vi "emi_Error Filter Single.vi"(1 "Action(No Error)":T2, 5 "Error Code":i32, 9 "error in (no error)":errorcluster, 12 "Filter(Error&Warning)":T1) -> (8 "Filter Triggered":bool, 10 "error out":errorcluster)   [LabVIEW 2011]
doc: "Filter error codes based on code(s). \n\nIf Code does not match, no action.\n\nIf code matches, the following is carried out:\nAction = No Error: Remove error.\nAction = Warning: Change from error to warning.\nAction = Error: Leave as Error.\nFilter Triggered is set to True.\n\nIf filtering both Warnings and errors, use bothe Error Filter.vi and Warning Filter.vi"
uses:
  emi_Error&Warning Filter Action.ctl
  _emi_Filter type.ctl
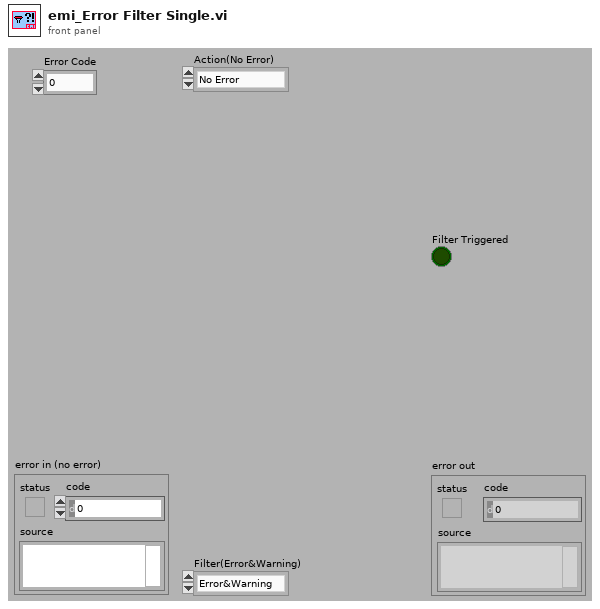
[diagram p1: front panel]
types:
  T1 = typedef "_emi_Filter type.ctl" = enum16{"Error&Warning", "Warning", "Error"}
  T2 = typedef "emi_Error&Warning Filter Action.ctl" = enum16{"No Error", "Warning", "Error"}
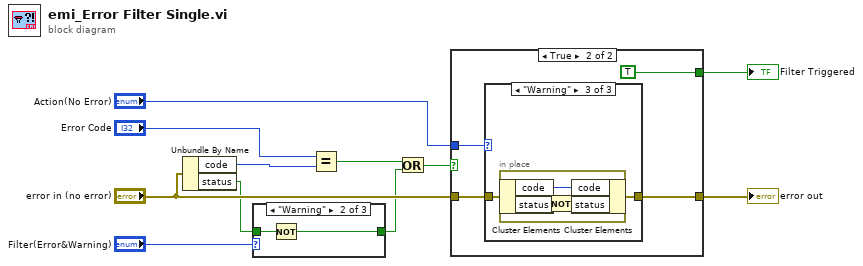
[diagram p0: block diagram]
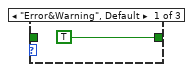
[diagram p2: hidden frame]
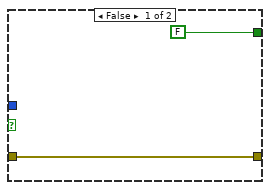
[diagram p4: hidden frame]
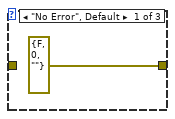
[diagram p5: hidden frame]
diagram:
  n1 = Unbundle By Name("error in (no error)") -> ("code"=w7:i32, "status"=w3:bool)
  n2 = case shown="\"Warning\"" "Filter(Error&Warning)" {
    tunnel: w3 -> [_ w14 w15]
    tunnel: [TRUE w13 w15] -> w2
    frame "Error&Warning", Default {
    }
    frame "Warning" {
      n3 = Not(x=w14) -> (.not. x?=w13:bool)
    }
    frame "Error" {
    }
  }
  n4 = Equal?(x="Error Code", y=w7) -> (x = y?=w6:bool)
  n5 = Or(x=w6, y=w2) -> (x .or. y?=w5:bool)
  n6 = case shown="True" w5 {
    tunnel: [w17 w21] -> w10
    tunnel: "error in (no error)" -> [w17 w20]
    tunnel: "Action(No Error)" -> [_ w19]
    tunnel: [FALSE TRUE] -> w8
    frame False {
    }
    frame True {
      n7 = case shown="\"Warning\"" w19 {
        tunnel: [errorcluster {"status"=FALSE, "code"=0, "source"=""} ("error IO") w23 w24] -> w21
        tunnel: w20 -> [_ w23 w25]
        frame "No Error", Default {
        }
        frame "Error" {
        }
        frame "Warning" {
          n8 = in-place {
            n9 = in-place-cluster #1(w25) -> ("code"=w28:i32, "status"=w26:bool)
            n10 = Not(x=w26) -> (.not. x?=w27:bool)
            n11 = in-place-cluster #1("code"=w28, "status"=w27) -> (w24:errorcluster)
          }
        }
      }
    }
  }
  "error out" <- w10
  "Filter Triggered" <- w8
